vi "Open_Instr.vi"(8 "error in (no error)":errorcluster caption="entrée d'erreur (pas d'erreur)", 11 "Class Firebase Altyor en entrée":refnum<class "Class Instrument Firebase Altyor.lvclass">) -> (0 "error out":errorcluster caption="sortie d'erreur", 3 "Class  Firebase Altyor en sortie":refnum<class "Class Instrument Firebase Altyor.lvclass">)   [LabVIEW 2020, in "Library Instrument & Equipement.lvlib" / "Library Instruments.lvlib" / "Class Instrument Firebase Altyor.lvclass"]
uses:
  Class Instrument Firebase Altyor.lvclass
  Commun VI/TypeDef/Bench Type.ctl
  Firebase/Source/Firebase AssembledProducts/Firebase AssembledProducts.lvclass
  Class Instrument Firebase Altyor.lvclass/Class Instrument Firebase Altyor.ctl
  Firebase/Source/Firebase Altyor/Firebase Altyor.lvclass
  C:/Users/ngarcin/OneDrive - Altyor/Standard TB/Class/Firebase/Source/Firebase Driver/Firebase Driver.lvclass
  Instrument (Default)/Class Instrument (Default).lvclass
  Firebase/Source/Firebase PCBA/Firebase Benches.lvclass
  Commun VI/TypeDef/Liste Error.ctl
  Firebase/Source/Firebase Benches P2193/Firebase Benches P2193.lvclass
  Commun VI/Library Commun.lvlib
  C:/Users/ngarcin/OneDrive - Altyor/Standard TB/Class/Firebase/Source/Firebase Altyor/Firebase Altyor.lvclass
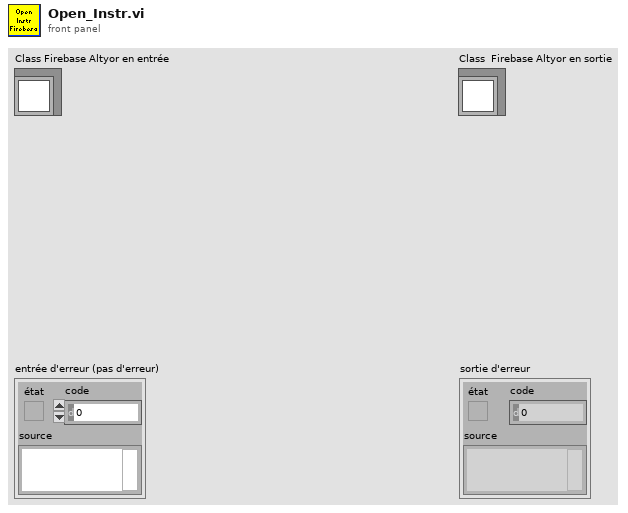
[diagram p1: front panel]
types:
  T1 = typedef "Library Commun.lvlib/Bench Type.ctl" = enum16{"Bench PCBA", "Bench Camera", "Bench Assembly", "Bench PCBA P2193"}
  T2 = typedef "Library Commun.lvlib/Liste Error.ctl" = enum16{"Firebase Driver - Get Document", "Firebase Driver - Get Document With Where", "Firebase Driver - Delete Document", "Firebase Driver - Set Document", "Firebase Driver - Update Document", "Firebase Altyor - Search Document Bench", "Firebase Altyor - Class Not in Firebase", "Spectrum_Analyser - Timeout", "Relay Board - Qty Relay", "DIO - Pb Funtion", "Power_Supply - Peripherical not find", "Mutimeter - Peripherical not find", "Instrument - Function Not Used", "Instrument - Instrument name not specified", "Instrument - Allready Initialised", "Instrument - TimeOut", "Instrument - the instrument must be Initialise before", "Instrument - Frame Not received", "Instrument - Frame Nok", "Test - Initialise the File_for_Save", "Test - Timeout", "Test - Cmd Error", "FGV - Variable ", "BDD FireBase - Define Class", "SN - Class Not Define"}
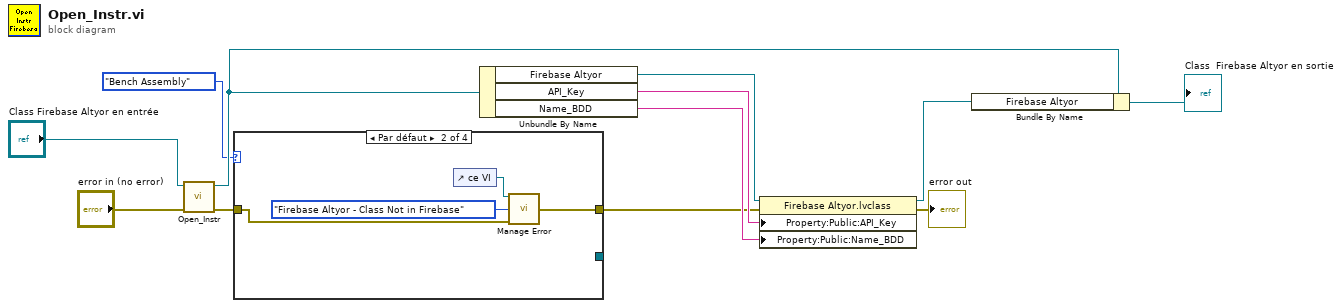
[diagram p0: block diagram]
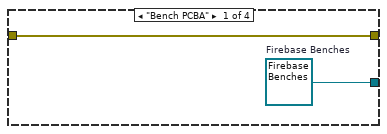
[diagram p2: hidden frame]
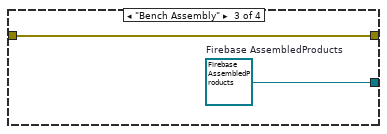
[diagram p3: hidden frame]
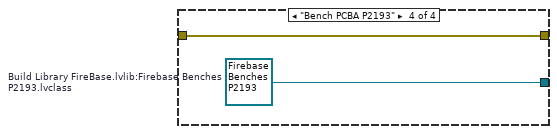
[diagram p4: hidden frame]
diagram:
  n1 = call-parent "Open_Instr.vi"("error in (no error)"="error in (no error)", "Class Multimeter (Default) en entrée"="Class Firebase Altyor en entrée") -> ("error out"=w9:errorcluster, "Class Multimeter (Default) en sortie"=w10:refnum<class "Class Instrument Firebase Altyor.lvclass">)  [unwired: 8 in]
  n2 = case shown="Par défaut" Bench_Type."Bench Assembly" ("Bench Type") {
    tunnel: [w14 _ w20 w22] -> _
    tunnel: w9 -> [w13 w15 w19 w21]
    tunnel: [w13 w16 w19 w21] -> w8
    frame "Bench PCBA" {
      w14 = refnum<class "Firebase Benches.lvclass"> refnum  # Firebase Benches
    }
    frame Default {
      n3 = control-ref of="ce VI"() -> (w18:refnum<vi>)
      n4 = call "Manage Error.vi"("VI in Error"=w18, "Code Erreur"=Liste_Error."Firebase Altyor - Class Not in Firebase", "error in (no error)"=w15) -> ("error out"=w16:errorcluster)  [unwired: 12 in]
    }
    frame "Bench Assembly" {
      w20 = refnum<class "Firebase AssembledProducts.lvclass"> refnum  # Firebase AssembledProducts
    }
    frame "Bench PCBA P2193" {
      w22 = refnum<class "Firebase Benches P2193.lvclass"> refnum  # Build Library FireBase.lvlib:Firebase Benches P2193.lvclass
    }
  }
  n5 = Unbundle By Name(w10) -> ("Firebase Altyor"=w1:refnum<class "Firebase Altyor.lvclass">, "API_Key"=w12:string, "Name_BDD"=w11:string)
  n6 = property class="Firebase Altyor.lvclass"(reference=w1, error in=w8, "Property:Public:API_Key"=w12, "Property:Public:Name_BDD"=w11) -> (reference out=w3:refnum<class "Firebase Altyor.lvclass">, error out=→"error out":errorcluster)
  n7 = Bundle By Name(cluster=w10, "Firebase Altyor"=w3) -> (→"Class  Firebase Altyor en sortie":refnum<class "Class Instrument Firebase Altyor.lvclass">)
